vi "Get Element Types.vi"(8 "error in (no error)":errorcluster, 11 "JSON Array in":refnum<class "JSON Array.lvclass">) -> (0 "error out":errorcluster, 1 "single type?":bool, 2 "types":T1[](array[typedef]), 3 "JSON Array out":refnum<class "JSON Array.lvclass">)   [LabVIEW 2015, in "LVJSON.lvlib" / "JSON Array.lvclass"]
uses:
  JSON Array.lvclass
  JSON Types.ctl
  JSON Array.lvclass/JSON Array.ctl
  JSON Datatype/JSON Null.lvclass
  LVJSON.lvlib
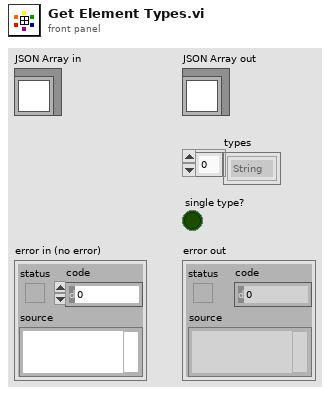
[diagram p1: front panel]
types:
  T1 = typedef "LVJSON.lvlib/JSON Types.ctl" = enum16{"String", "Numeric", "Boolean", "NULL", "Object", "Array"}
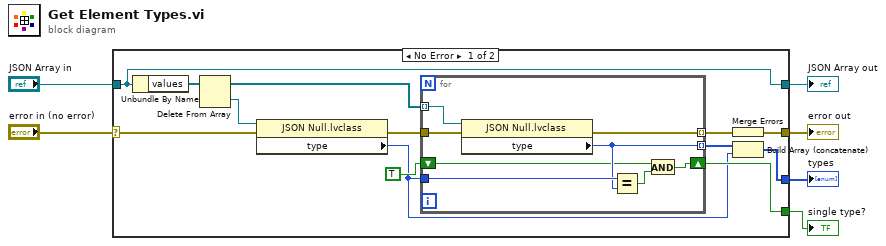
[diagram p0: block diagram]
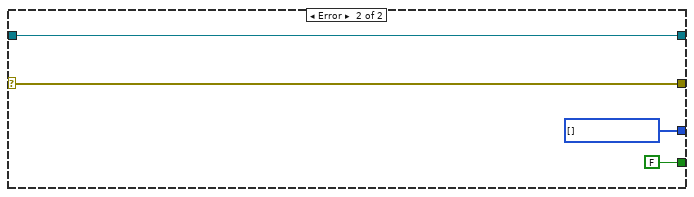
[diagram p2: hidden frame]
diagram:
  n1 = case shown="No Error" "error in (no error)" {
    selector: "error in (no error)" -> [w10 w31]
    tunnel: [w7 w31] -> w5
    tunnel: [w19 w30] -> w3
    tunnel: "JSON Array in" -> [w19 w30]
    tunnel: [w13 w29] -> w2
    tunnel: [w15 FALSE] -> w1
    frame No Error {
      n2 = Unbundle By Name(w19) -> ("values"=w11:refnum<class "JSON Null.lvclass">[])
      n3 = Delete From Array(array=w11) -> (deleted portion=w18:refnum<class "JSON Null.lvclass">, array with subset deleted=w17:refnum<class "JSON Null.lvclass">[])  [unwired: 2 in]
      n4 = property class="JSON Null.lvclass"(reference=w18, error in=w10) -> (error out=w9:errorcluster, "type"=w12:T1)  [unwired: 1 out]
      n5 = for {
        tunnel: w17 -> [w27] mode=indexing
        tunnel: [w25] -> w14 mode=indexing
        tunnel: w12 -> [w26]
        shift-right: [w22] -> w15
        shift-left: TRUE -> [w23]
        tunnel: w9 -> [w21]
        tunnel: [w20] -> w8 mode=indexing
        n6 = property class="JSON Null.lvclass"(reference=w27, error in=w21) -> (error out=w20:errorcluster, "type"=w25:T1)  [unwired: 1 out]
        n7 = Equal?(x=w26, y=w25) -> (x = y?=w24:bool)
        n8 = And(x=w23, y=w24) -> (x .and. y?=w22:bool)
      }
      n9 = Merge Errors(w8) -> (w7:errorcluster)
      n10 = Build Array (concatenate)(w14, w12) -> (w13:T1[])
    }
    frame Error {
      w29 = T1[] [] items=["String", "Numeric", "Boolean", "NULL", "Object", "Array"]
    }
  }
  "error out" <- w5
  "JSON Array out" <- w3
  "types" <- w2
  "single type?" <- w1
